vi "handleSettings.vi"(8 "error in (no error)":errorcluster, 10 "Path":path, 11 "ICCameraController in":refnum<class "ICCameraController.lvclass">) -> (0 "error out":errorcluster, 3 "ICCameraController out":refnum<class "ICCameraController.lvclass">)   [LabVIEW 2011, in "Hardware.lvlib" / "Channels.lvlib" / "ICCameraController.lvclass"]
doc: "Override this method in a subclass to load specific settings for the camera being used."
uses:
  ICCameraController.lvclass
  CameraEventsManager/CameraEventsManger.lvclass
  CameraAcquisitor.lvclass
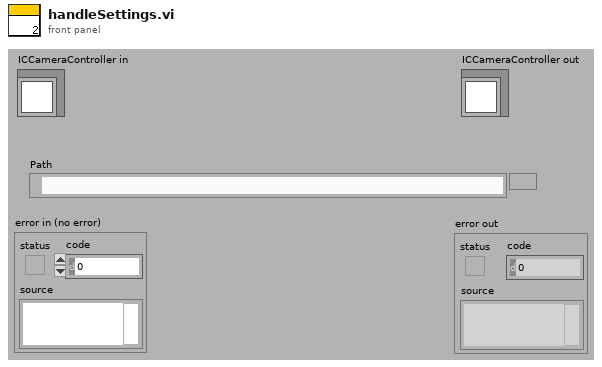
[diagram p1: front panel]
types:
  T1 = cluster{"settingsFrontEndEvents":cluster{"loadSettingsFromPath":refnum<user-event>, "lookUpElementEvent":refnum<user-event>, "saveSettings":refnum<user-event>, "loadSettings":refnum<user-event>, "close":refnum<user-event>, "replaceElement":refnum<user-event>, "findParentNodes":refnum<user-event>, "createNode":refnum<user-event>}, "settingBackEndEvents":cluster{"defaultSettingsPathRequest":refnum<user-event>, "searchResultEvent":refnum<user-event>, "settingsSaved":refnum<user-event>, "settingsLoaded":refnum<user-event>, "foundParentNode":refnum<user-event>}}
  T2 = cluster{"loadSettingsFromPath":refnum<user-event>, "lookUpElementEvent":refnum<user-event>, "saveSettings":refnum<user-event>, "loadSettings":refnum<user-event>, "close":refnum<user-event>, "replaceElement":refnum<user-event>, "findParentNodes":refnum<user-event>, "createNode":refnum<user-event>}
  T3 = cluster{"defaultSettingsPathRequest":refnum<user-event>, "searchResultEvent":refnum<user-event>, "settingsSaved":refnum<user-event>, "settingsLoaded":refnum<user-event>, "foundParentNode":refnum<user-event>}
  T4 = enum16{"Number", "String", "NumberArray", "StringArray", "xmlNode"}
  T5 = cluster{string, string, "typeEnum":enum16{"Number", "String", "NumberArray", "StringArray", "xmlNode"}}
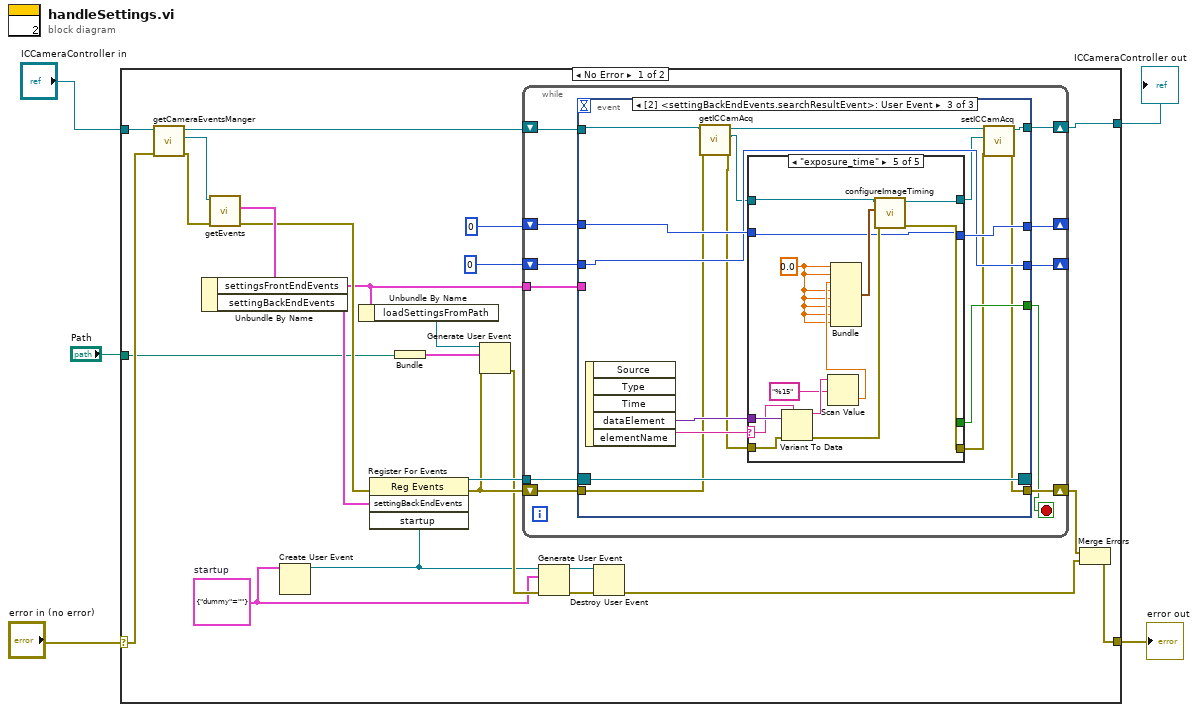
[diagram p0: block diagram]
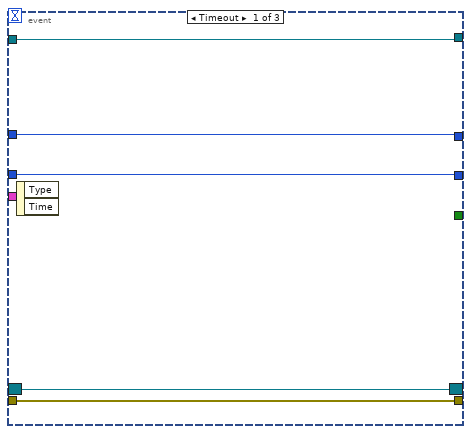
[diagram p2: hidden frame]
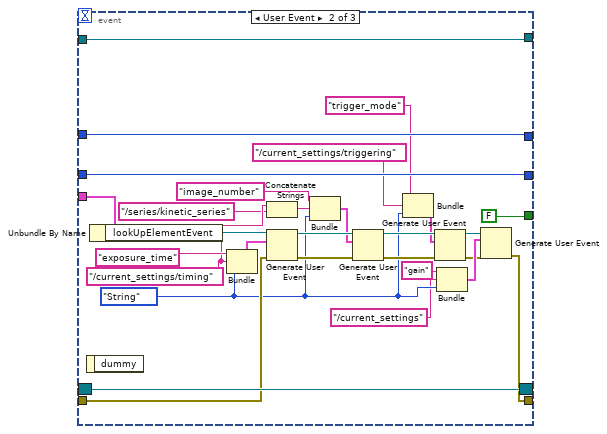
[diagram p3: hidden frame]
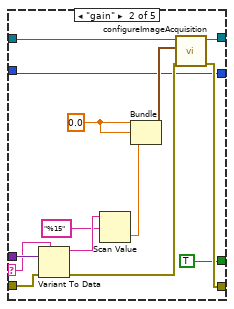
[diagram p5: hidden frame]
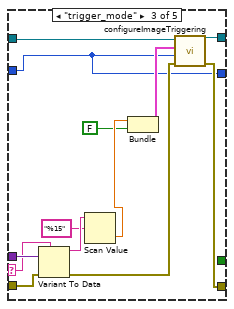
[diagram p6: hidden frame]
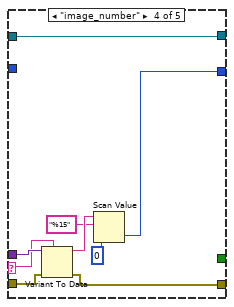
[diagram p7: hidden frame]
diagram:
  n1 = case shown="No Error" "error in (no error)" {
    selector: "error in (no error)" -> [w29 w144]
    tunnel: "ICCameraController in" -> [w30 w145]
    tunnel: [w7 w144] -> w3
    tunnel: [w10 w145] -> w2
    tunnel: "Path" -> [w19 _]
    frame No Error {
      w12 = cluster{"dummy":string} {"dummy"=""}  # startup
      n2 = call-dynamic "getCameraEventsManger.vi"("error in (no error)"=w29, "CameraController.lvclass in"=w30) -> ("error out"=w26:errorcluster, "Hardware:Channels.lvlib:CameraEventsManger.lvclass"=w28:refnum<class "CameraEventsManger.lvclass">, "CameraController.lvclass out"=w11:refnum<class "ICCameraController.lvclass">)  [unwired: 7 in]
      n3 = call-dynamic "getEvents.vi"("error in (no error)"=w26, "CameraEventsManger in"=w28) -> ("error out"=w24:errorcluster, "settingsEvents"=w27:T1)  [unwired: 5 in, 3 out]
      n4 = Unbundle By Name(w27) -> ("settingsFrontEndEvents"=w14:T2, "settingBackEndEvents"=w25:T3)
      n5 = Create User Event(user event datatype=w12) -> (user event=w17:refnum<user-event>)  [unwired: 1 in, 1 out]
      n6 = Unbundle By Name(w14) -> ("loadSettingsFromPath"=w22:refnum<user-event>)
      n7 = register-events(error in=w24, w25, w17) -> (reference out=w23:refnum<event-registration>, error out=w21:errorcluster)  [unwired: 1 in]
      n8 = Bundle("Path"=w19) -> (w20:cluster{"Path":path})  [unwired: 1 in]
      n9 = Generate User Event(user event=w22, event data cluster=w20, error in=w21) -> (error out=w18:errorcluster)  [unwired: 1 out]
      n10 = while {
        tunnel: w23 -> [w41]
        shift-right: [w39] -> w9
        shift-left: w21 -> [w40]
        tunnel: w14 -> [w38]
        shift-right: [w35] -> _
        shift-left: 0 -> [w37]
        shift-right: [w33] -> w10
        shift-left: w11 -> [w34]
        shift-right: [w32] -> _
        shift-left: 0 -> [w31]
        stop <- w36 stop-if-true
        n11 = event shown="[2] <settingBackEndEvents.searchResultEvent>: User Event" {
          selector: w41 -> [w45 w75 w91]
          dyn-events: [w45 w75 w91] -> _
          timeout: _ -> [_ _ _]
          tunnel: w40 -> [w46 w67 w83]
          tunnel: [w46 w66 w77] -> w39
          tunnel: w38 -> [_ w74 _]
          tunnel: w37 -> [w44 w71 w86]
          tunnel: [_ FALSE w85] -> w36
          tunnel: [w44 w71 w86] -> w35
          tunnel: w34 -> [w43 w70 w84]
          tunnel: [w43 w70 w76] -> w33
          tunnel: [w42 w64 w88] -> w32
          tunnel: w31 -> [w42 w64 w87]
          event Timeout {
            n12 = event-data() -> ()  [unwired: 1 in, 2 out]
          }
          event User Event {
            w54 = T4."String" ("typeEnum")
            w51 = "/current_settings/timing"
            n13 = event-data() -> ()  [unwired: 1 in, 1 out]
            n14 = Unbundle By Name(w74) -> ("lookUpElementEvent"=w73:refnum<user-event>)
            n15 = Bundle("exposure_time", w51, "typeEnum"=w54) -> (w57:T5)  [unwired: 1 in]
            n16 = Concatenate Strings(w51, "/series/kinetic_series") -> (w49:string)
            n17 = Generate User Event(user event=w73, event data cluster=w57, error in=w67) -> (user event out=w63:refnum<user-event>, error out=w60:errorcluster)
            n18 = Bundle("image_number", w49, "typeEnum"=w54) -> (w55:T5)  [unwired: 1 in]
            n19 = Generate User Event(user event=w63, event data cluster=w55, error in=w60) -> (user event out=w62:refnum<user-event>, error out=w61:errorcluster)
            n20 = Bundle("trigger_mode", "/current_settings/triggering", "typeEnum"=w54) -> (w53:T5)  [unwired: 1 in]
            n21 = Generate User Event(user event=w62, event data cluster=w53, error in=w61) -> (user event out=w58:refnum<user-event>, error out=w59:errorcluster)
            n22 = Bundle("gain", "/current_settings", "typeEnum"=w54) -> (w68:T5)  [unwired: 1 in]
            n23 = Generate User Event(user event=w58, event data cluster=w68, error in=w59) -> (error out=w66:errorcluster)  [unwired: 1 out]
          }
          event User Event {
            n24 = event-data() -> ("dataElement"=w89:variant, "elementName"=w90:string)  [unwired: 1 in, 3 out]
            n25 = call-dynamic "getICCamAcq.vi"("error in (no error)"=w83, "ICCameraController in"=w84) -> ("error out"=w82:errorcluster, "ICCameraAcquisitor"=w81:refnum<class "ICCameraAcquisitor.lvclass">, "ICCameraController out"=w80:refnum<class "ICCameraController.lvclass">)  [unwired: 7 in]
            n26 = case shown="\"exposure_time\"" w90 {
              selector: w90 -> [_ w105 w118 w128 w142]
              tunnel: w89 -> [_ w106 w119 w129 w143]
              tunnel: w82 -> [w93 w104 w117 w127 w141]
              tunnel: [w93 w98 w114 w122 w134] -> w78
              tunnel: w81 -> [w94 w101 w116 w130 w132]
              tunnel: [w94 w97 w115 w130 w131] -> w79
              tunnel: [w92 w96 w109 w124 w133] -> w88
              tunnel: w87 -> [w92 w96 w109 _ w133]
              tunnel: [_ TRUE _ _ _] -> w85
              frame Default {
              }
              frame "gain" {
                w103 = 0.0
                n27 = Variant To Data(error in=w104, type=w105, Variant=w106) -> (data=w108:string, error out=w99:errorcluster)
                n28 = Scan Value(string=w108, format string="%15") -> (value=w102:dbl)  [unwired: 1 in, 1 out]
                n29 = Bundle(w103, w103, w102) -> (w100:cluster{dbl, dbl, dbl})  [unwired: 1 in]
                n30 = call "configureImageAcquisition.vi"("error in (no error)"=w99, "Mode"=w100, "CameraAcquisitor in"=w101) -> ("error out"=w98:errorcluster, "CameraAcquisitor out"=w97:refnum<class "ICCameraAcquisitor.lvclass">)  [unwired: 7 in]
              }
              frame "trigger_mode" {
                n31 = Variant To Data(error in=w117, type=w118, Variant=w119) -> (data=w121:string, error out=w111:errorcluster)
                n32 = Scan Value(string=w121, format string="%15") -> (value=w113:dbl)  [unwired: 1 in, 1 out]
                n33 = Bundle(w113, FALSE) -> (w110:cluster{dbl, bool})  [unwired: 1 in]
                n34 = call "configureImageTriggering.vi"("error in (no error)"=w111, "Number of Images"=w109, "Triggering"=w110, "CameraAcquisitor in"=w116) -> ("error out"=w114:errorcluster, "CameraAcquisitor out"=w115:refnum<class "ICCameraAcquisitor.lvclass">)  [unwired: 6 in]
              }
              frame "image_number" {
                n35 = Variant To Data(error in=w127, type=w128, Variant=w129) -> (data=w126:string, error out=w122:errorcluster)
                n36 = Scan Value(string=w126, format string="%15", default (0 dbl)=0) -> (value=w124:i32)  [unwired: 1 out]
              }
              frame "exposure_time" {
                w137 = 0.0
                n37 = Variant To Data(error in=w141, type=w142, Variant=w143) -> (data=w140:string, error out=w135:errorcluster)
                n38 = Scan Value(string=w140, format string="%15") -> (value=w138:dbl)  [unwired: 1 in, 1 out]
                n39 = Bundle(w137, w137, w138, w137, w137, w137, w137, w137) -> (w136:cluster{dbl, dbl, dbl, dbl, dbl, dbl, dbl, dbl})  [unwired: 1 in]
                n40 = call "configureImageTiming.vi"("error in (no error)"=w135, "Timing"=w136, "CameraAcquisitor in"=w132) -> ("error out"=w134:errorcluster, "CameraAcquisitor out"=w131:refnum<class "ICCameraAcquisitor.lvclass">)  [unwired: 7 in]
              }
            }
            n41 = call-dynamic "setICCamAcq.vi"("error in (no error)"=w78, "ICCameraAcquisitor"=w79, "ICCameraController in"=w80) -> ("error out"=w77:errorcluster, "ICCameraController out"=w76:refnum<class "ICCameraController.lvclass">)  [unwired: 7 in]
          }
        }
      }
      n42 = Generate User Event(user event=w17, event data cluster=w12, error in=w18) -> (user event out=w15:refnum<user-event>, error out=w16:errorcluster)
      n43 = Destroy User Event(user event=w15, error in=w16) -> (error out=w8:errorcluster)
      n44 = Merge Errors(w9, w8) -> (w7:errorcluster)
    }
    frame Error {
    }
  }
  "error out" <- w3
  "ICCameraController out" <- w2
